vi "Fetch Waveform Measurement.vi"(8 "error in (no error)":errorcluster, 9 "Measurement Function (0: Voltage Vpp)":u16(ring) items=["Voltage Vpp", "Voltage Max", "Voltage Min", "Amplitude", "Voltage TOP", "Voltage Base", "Voltage Average", "Voltage RMS", "Overshoot", "Preshoot", "Frequency", "Rise Time", "Fall Time", "Period", "Positive Width", "Negative Width", "Positive Duty", "Negative Duty"], 10 "Source (0: Channel 1)":u16(ring) items=["Channel 1", "Channel 2", "Channel 3", "Channel 4"], 11 "VISA resource name":refnum<visa-resource-name>) -> (0 "error out":errorcluster, 2 "Measured Value":dbl, 3 "VISA resource name out":refnum<visa-resource-name>)   [LabVIEW 2023, in "RIGOL DS1054Z Driver.lvlib"]
doc: "Fetch waveform measurement from oscilloscope.\n\n<B>Note:</B>\n Use this VI only with other low-level VIs."
uses:
  <instrlib>/RIGOL-DS1054Z-LabVIEW/RIGOL DS1054Z Driver.lvlib
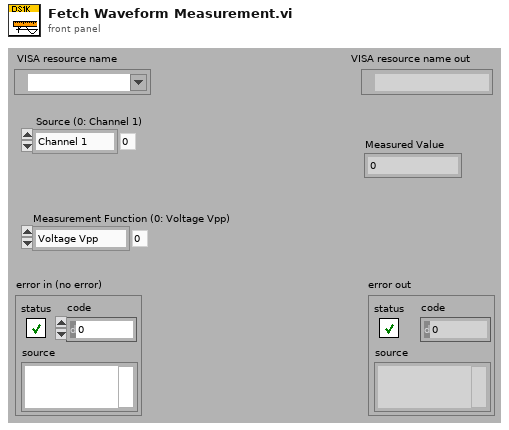
[diagram p1: front panel]
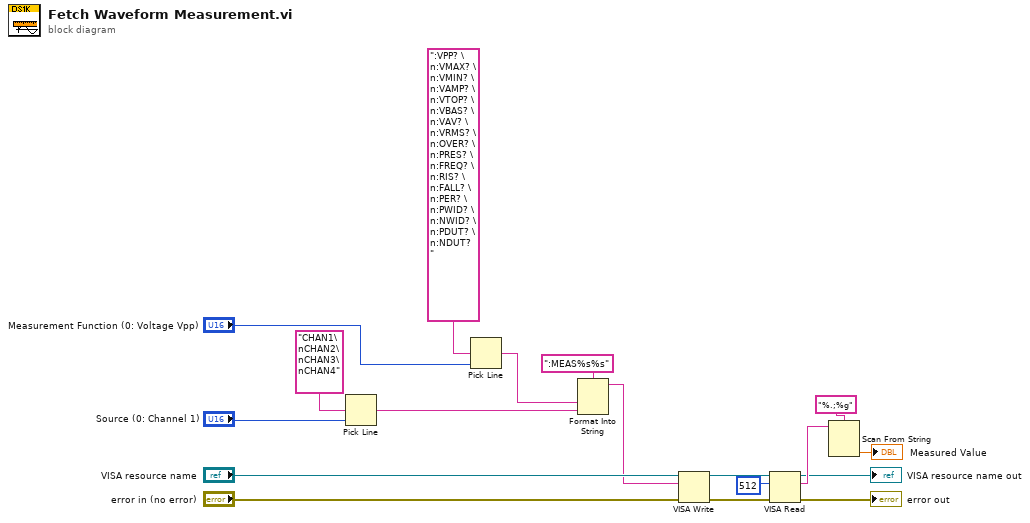
[diagram p0: block diagram]
diagram:
  n1 = Pick Line(multi-line string="CHAN1\nCHAN2\nCHAN3\nCHAN4", line index="Source (0: Channel 1)") -> (output string=w3:string)  [unwired: 1 out]
  n2 = Pick Line(multi-line string=":VPP? \n:VMAX? \n:VMIN? \n:VAMP? \n:VTOP? \n:VBAS? \n:VAV? \n:VRMS? \n:OVER? \n:PRES? \n:FREQ? \n:RIS? \n:FALL? \n:PER? \n:PWID? \n:NWID? \n:PDUT? \n:NDUT? ", line index="Measurement Function (0: Voltage Vpp)") -> (output string=w4:string)  [unwired: 1 out]
  n3 = Format Into String(format string=":MEAS%s%s" ("格式字符串"), w4, w3) -> (resulting string=w2:string)  [unwired: 2 in, 1 out]
  n4 = VISA Write(VISA resource name="VISA resource name", write buffer=w2, error in (no error)="error in (no error)") -> (VISA resource name out=w14:refnum<visa-resource-name>, error out=w15:errorcluster)  [unwired: 1 out]
  n5 = VISA Read(VISA resource name=w14, byte count=u32 512, error in (no error)=w15) -> (VISA resource name out=→"VISA resource name out":refnum<visa-resource-name>, read buffer=w10:string, error out=→"error out":errorcluster)  [unwired: 1 out]
  n6 = Scan From String(format string="%.;%g", input string=w10) -> (output 1=→"Measured Value":dbl)  [unwired: 2 in, 4 out]
